vi "子界面-查看某框.vi"(0 "框号":dbl format="%#_13g", 1 "框组":T3(array[cluster]), 2 "临界Z值":i32, 3 "反射图原始路径":path, 4 "临界面积百分比值":dbl, 5 "预先配置的灰度阈值":dbl, 6 "穿透图原始路径":path, 7 "部位信息":string[](array[string])=["", "34.500000", "32.500000", "1121", "34", "54.955926", "分层类", "不合格", ""], 12 "产品规格":cluster{"产品长度（周长）（mm）":dbl, "产品宽度（母线长）（mm）":dbl}) -> (14 "弥散类检测结果":string[][](table), 19 "分层类检测结果":string[][](table))   [LabVIEW 2018]
uses:
  <vilib>/vision/NI_Vision_Development_Module.lvlib
panel:
  in  "格式字符串 3":string="%f"
  in  "分隔符（'\\'代码显示） 2":string="\t"
  out "弥散和分层临界灰度值":i64
  out "弥散缺陷个数":i32
  out "分层缺陷个数":i32
  out "合格？ 弥散类":string="fencengThreshold"
  out "合格？分层类":string="fencengThreshold"
  in  "stop":bool caption="停止"
  out "?":T1(plugin-control)
  out "Threshold Image":T1(plugin-control)
  out "Threshold Image":T1(plugin-control)
  out "Threshold Image":T1(plugin-control)
  in  "Tab Control":T2
  out "穿透ROI":T1(plugin-control)
  out "Threshold Image":T1(plugin-control)
  out "?":T1(plugin-control)
  out "?":T1(plugin-control)
  out "Threshold Image":T1(plugin-control)
  out "Threshold Image":T1(plugin-control)
  out "弥散测量结果":dbl[][](array[numeric]) format="%.2f"
  out "?":string
  out "面积 (pixels)":i32
  in  "格式字符串 2":string="%f"
  in  "分隔符（'\\'代码显示）":string="\t"
  out "分层测量结果":dbl[][](array[numeric]) format="%.2f"
  out "缺陷初步分类的临界值":sgl format="%#.3f"
  # "所选区域信息"
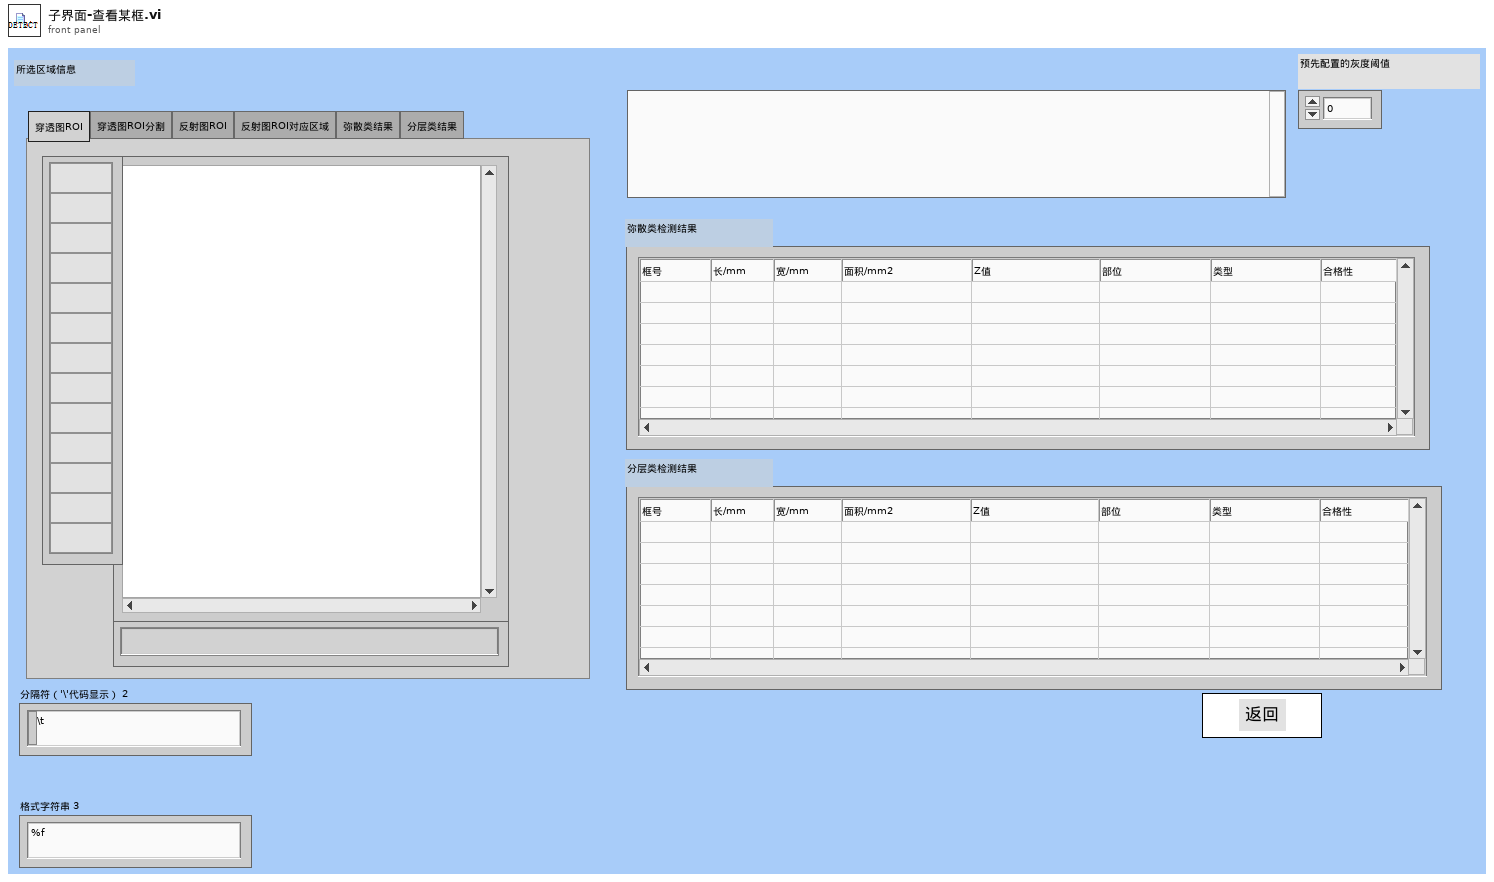
[diagram p1: front panel]
types:
  T1 = typedef "IMAQ Image.ctl" = refnum<image>
  T2 = typedef "控件 1.ctl" = enum32{"穿透图ROI", "穿透图ROI分割", "反射图ROI", "反射图ROI对应区域", "弥散类结果", "分层类结果"}
  T3 = cluster{"Global Rectangle":i32[], "Contours":cluster{"Contour Type":u32, "ROI Type":u32, "Points":i32[]}[]}[]
  T4 = typedef "Image Type" = u32
  T5 = typedef "Particle Parameters" = i32
  T6 = cluster{"Measurement Parameter":T5, "Range Lower Value":dbl, "Range Upper Value":dbl, "Range":bool, "Measurement Type":bool}[]
  T7 = cluster{"Global Rectangle":i32[], "Contours":cluster{"Contour Type":u32, "ROI Type":u32, "Points":i32[]}[]}
  T8 = cluster{"histogram":u32[], "Minimal Value":sgl, "Maximal Value":sgl, "Starting Value":sgl, "Interval Width":sgl, "Mean Value":sgl, "Standard  Variation":sgl, "Area (pixels)":i32}
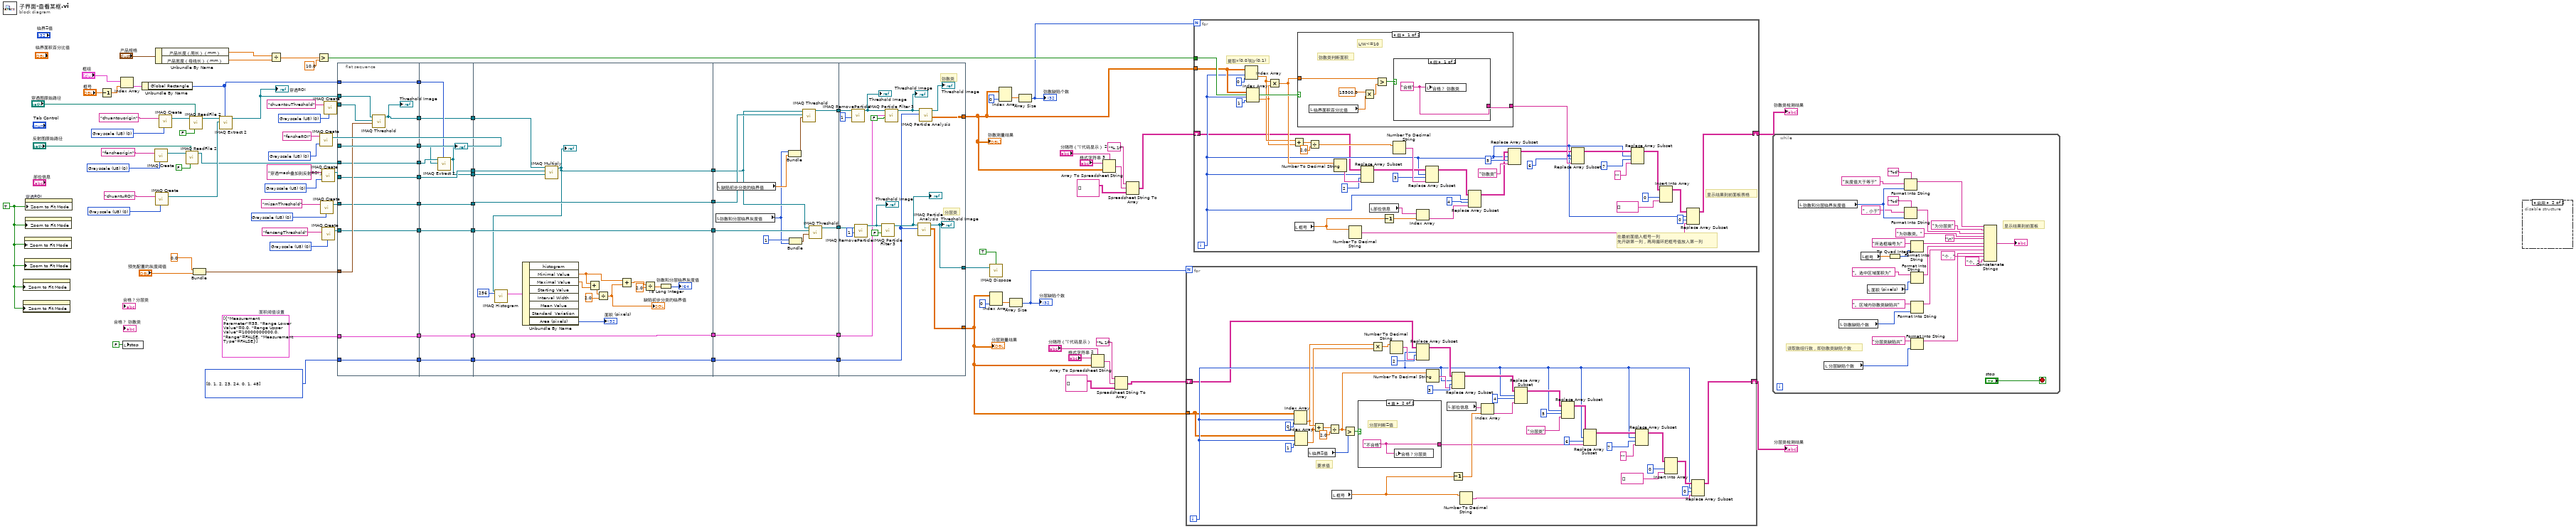
[diagram p0: block diagram]
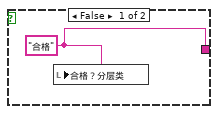
[diagram p2: hidden frame]
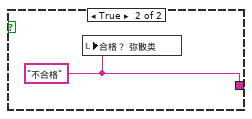
[diagram p3: hidden frame]
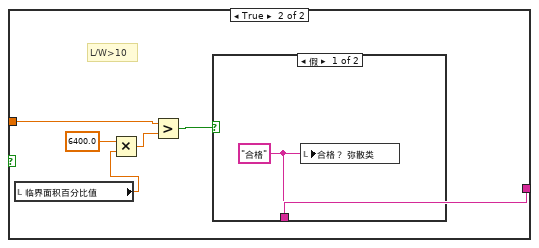
[diagram p4: hidden frame]
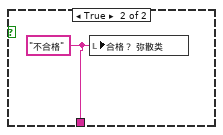
[diagram p5: hidden frame]
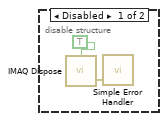
[diagram p6: hidden frame]
diagram:
  w62 = T4 0 items=["Grayscale (U8)", "Grayscale (I16)", "Grayscale (SGL)", "Complex (CSG)", "RGB (U32)", "HSL (U32)", "RGB (U64)", "Grayscale (U16)"] ("Image Type")
  w63 = T4 0 items=["Grayscale (U8)", "Grayscale (I16)", "Grayscale (SGL)", "Complex (CSG)", "RGB (U32)", "HSL (U32)", "RGB (U64)", "Grayscale (U16)"] ("Image Type")
  w64 = T4 0 items=["Grayscale (U8)", "Grayscale (I16)", "Grayscale (SGL)", "Complex (CSG)", "RGB (U32)", "HSL (U32)", "RGB (U64)", "Grayscale (U16)"] ("Image Type")
  w68 = T4 0 items=["Grayscale (U8)", "Grayscale (I16)", "Grayscale (SGL)", "Complex (CSG)", "RGB (U32)", "HSL (U32)", "RGB (U64)", "Grayscale (U16)"] ("Image Type")
  w72 = T4 0 items=["Grayscale (U8)", "Grayscale (I16)", "Grayscale (SGL)", "Complex (CSG)", "RGB (U32)", "HSL (U32)", "RGB (U64)", "Grayscale (U16)"] ("Image Type")
  w22 = i32[] [0, 1, 2, 23, 24, 0, 1, 48] items=["Bounding Rect Width", "Bounding Rect Height", "Area"] ("Pixel Measurements")
  w27 = T6 [{"Measurement Parameter"=35, "Range Lower Value"=0.0, "Range Upper Value"=10000000000.0, "Range"=FALSE, "Measurement Type"=FALSE}]  # 面积阈值设置
  w86 = T4 0 items=["Grayscale (U8)", "Grayscale (I16)", "Grayscale (SGL)", "Complex (CSG)", "RGB (U32)", "HSL (U32)", "RGB (U64)", "Grayscale (U16)"] ("Image Type")
  w55 = T4 0 items=["Grayscale (U8)", "Grayscale (I16)", "Grayscale (SGL)", "Complex (CSG)", "RGB (U32)", "HSL (U32)", "RGB (U64)", "Grayscale (U16)"] ("Image Type")
  w90 = T4 0 items=["Grayscale (U8)", "Grayscale (I16)", "Grayscale (SGL)", "Complex (CSG)", "RGB (U32)", "HSL (U32)", "RGB (U64)", "Grayscale (U16)"] ("Image Type")
  w98 = TRUE ("Zoom to Fit Mode")
  n1 = property class="ImageControl"("Zoom to Fit Mode"=w98) -> ()  [unwired: 2 in, 2 out]
  n2 = property class="ImageControl"("Zoom to Fit Mode"=w98) -> ()  [unwired: 2 in, 2 out]
  n3 = property class="ImageControl"("Zoom to Fit Mode"=w98) -> ()  [unwired: 2 in, 2 out]
  n4 = property class="ImageControl"("Zoom to Fit Mode"=w98) -> ()  [unwired: 2 in, 2 out]
  n5 = property class="ImageControl"("Zoom to Fit Mode"=w98) -> ()  [unwired: 2 in, 2 out]
  n6 = property on="穿透ROI" class="ImageControl"("Zoom to Fit Mode"=w98) -> ()  [unwired: 2 in, 2 out]
  n7 = Decrement(x="框号") -> (x-1=w92:dbl)
  n8 = Index Array(array="框组", index=w92) -> (element=w93:T7)
  n9 = local write "stop"(FALSE ("stop")) -> ()
  n10 = Unbundle By Name(w93) -> ("Global Rectangle"=w54:i32[])
  n11 = call "IMAQ Create"("Image Name"="fansheorigin", "Image Type"=w68) -> ("New Image"=w67:T1)  [unwired: 3 in, 1 out]
  n12 = call "IMAQ Create"("Image Name"="chuantuROI", "Image Type"=w72) -> ("New Image"=w71:T1)  [unwired: 3 in, 1 out]
  n13 = Unbundle By Name("产品规格") -> ("产品长度（周长）（mm）"=w80:dbl, "产品宽度（母线长）（mm）"=w79:dbl)
  n14 = call "IMAQ Create"("Image Name"="chuantouorigin", "Image Type"=w90) -> ("New Image"=w74:T1)  [unwired: 3 in, 1 out]
  n15 = call "IMAQ ReadFile 2"("Use File Path Image Type"=FALSE, "File Path"="反射图原始路径", "Image"=w67) -> ("Image Out"=w50:T1)  [unwired: 4 in, 4 out]
  n16 = call "IMAQ ReadFile 2"("Use File Path Image Type"=FALSE, "File Path"="穿透图原始路径", "Image"=w74) -> ("Image Out"=w75:T1)  [unwired: 4 in, 4 out]
  n17 = Bundle(0.0, "预先配置的灰度阈值"="预先配置的灰度阈值") -> (w17:cluster{dbl, "预先配置的灰度阈值":dbl})  [unwired: 1 in]
  n18 = call "IMAQ Extract 2"("Optional Rectangle"=w54, "Image Dst"=w71, "Image Src"=w75) -> ("Image Dst Out"=w52:T1)  [unwired: 7 in, 1 out]
  "穿透ROI" <- w52
  n19 = Divide(x=w80, y=w79) -> (x/y=w83:dbl)
  n20 = Greater?(x=w83, y=10.0) -> (0:w78:bool)
  n21 = call "IMAQ Create"("Image Name"="fansheROI", "Image Type"=w55) -> ("New Image"=w51:T1)  [unwired: 3 in, 1 out]
  n22 = call "IMAQ Create"("Image Name"="misanThreshold", "Image Type"=w62) -> ("New Image"=w37:T1)  [unwired: 3 in, 1 out]
  n23 = call "IMAQ Create"("Image Name"="穿透mask叠加到反射ROI上", "Image Type"=w86) -> ("New Image"=w45:T1)  [unwired: 3 in, 1 out]
  n24 = call "IMAQ Create"("Image Name"="fencengThreshold", "Image Type"=w63) -> ("New Image"=w35:T1)  [unwired: 3 in, 1 out]
  n25 = call "IMAQ Create"("Image Name"="chuantouThreshold", "Image Type"=w64) -> ("New Image"=w53:T1)  [unwired: 3 in, 1 out]
  n26 = flat-sequence {
    tunnel: w54 -> [w110]
    tunnel: w53 -> [w109]
    tunnel: w52 -> [w108]
    tunnel: w17 -> [w107]
    tunnel: w51 -> [w106]
    tunnel: w50 -> [w105]
    tunnel: [w110] -> w49
    tunnel: [w106] -> w48
    tunnel: [w105] -> w47
    tunnel: [w104] -> w46
    tunnel: w45 -> [w104]
    tunnel: [w103] -> w42
    tunnel: w37 -> [w102]
    tunnel: [w102] -> w39
    tunnel: [w101] -> w36
    tunnel: w35 -> [w101]
    tunnel: [w100] -> w28
    tunnel: w27 -> [w100]
    tunnel: [w99] -> w23
    tunnel: w22 -> [w99]
    tunnel: w49 -> [w120]
    tunnel: w48 -> [w111]
    tunnel: w47 -> [w112]
    tunnel: w46 -> [w119]
    tunnel: [w119] -> w44
    tunnel: [w118] -> w43
    tunnel: w42 -> [w118]
    tunnel: [w117] -> w41
    tunnel: w39 -> [w116]
    tunnel: [w116] -> w38
    tunnel: w36 -> [w115]
    tunnel: [w115] -> w34
    tunnel: w28 -> [w114]
    tunnel: [w114] -> w26
    tunnel: w23 -> [w113]
    tunnel: [w113] -> w21
    tunnel: w44 -> [w140]
    tunnel: w43 -> [w139]
    tunnel: w41 -> [w138]
    tunnel: [w137] -> w40
    tunnel: w38 -> [w137]
    tunnel: w34 -> [w136]
    tunnel: [w136] -> w33
    tunnel: [w131] -> w32
    tunnel: w26 -> [w130]
    tunnel: [w130] -> w25
    tunnel: w21 -> [w129]
    tunnel: [w129] -> w20
    tunnel: w40 -> [w152]
    tunnel: w33 -> [w151]
    tunnel: w32 -> [w150]
    tunnel: [w149] -> w30
    tunnel: [w148] -> w29
    tunnel: w25 -> [w147]
    tunnel: [w147] -> w24
    tunnel: w20 -> [w146]
    tunnel: [w146] -> w19
    tunnel: [w163] -> w3
    tunnel: [w158] -> w11
    tunnel: [w157] -> w31
    tunnel: w30 -> [w156]
    tunnel: w29 -> [w155]
    tunnel: w24 -> [w154]
    tunnel: w19 -> [w153]
    frame #0 {
      n27 = call "IMAQ Threshold"("Range"=w107, "Image Dst"=w109, "Image Src"=w108) -> ("Image Dst Out"=w103:T1)  [unwired: 3 in, 5 out]
      "Threshold Image" <- w103
    }
    frame #1 {
      n28 = call "IMAQ Extract 2"("Optional Rectangle"=w120, "Image Dst"=w111, "Image Src"=w112) -> ("Image Dst Out"=w117:T1)  [unwired: 7 in, 1 out]
      "?" <- w117
    }
    frame #2 {
      n29 = call "IMAQ Multiply"("Image Src A"=w139, "Image Dst"=w140, "Image Src B"=w138) -> ("Image Dst Out"=w131:T1)  [unwired: 4 in, 1 out]
      "?" <- w131
      n30 = call "IMAQ Histogram"("Number of Classes"=256, "Image"=w131) -> ("Histogram Report"=w134:T8)  [unwired: 8 in, 1 out]
      n31 = Unbundle By Name(w134) -> ("Minimal Value"=w123:sgl, "Maximal Value"=w125:sgl, "Area (pixels)"=→"面积 (pixels)":i32)  [unwired: 5 out]
      n32 = Add(x=w123, y=w125) -> (x+y=w124:sgl)
      n33 = Divide(x=w124, y=sgl 2.0) -> (x/y=w122:sgl)
      "缺陷初步分类的临界值" <- w122
      n34 = Add(x=w123, y=w122) -> (x+y=w121:sgl)
      n35 = Divide(x=w121, y=sgl 2.0) -> (x/y=w126:sgl)
      n36 = To Long Integer(number=w126) -> (32bit integer=→"弥散和分层临界灰度值":i32)
    }
    frame #3 {
      n37 = local read "弥散和分层临界灰度值"() -> (w142:i64)
      n38 = local read "缺陷初步分类的临界值"() -> (w144:sgl)
      n39 = Bundle("弥散和分层临界灰度值"=w142, "缺陷初步分类的临界值"=w144) -> (w145:cluster{"弥散和分层临界灰度值":i64, "缺陷初步分类的临界值":sgl})  [unwired: 1 in]
      n40 = Bundle(1, "弥散和分层临界灰度值"=w142) -> (w141:cluster{i32, "弥散和分层临界灰度值":i64})  [unwired: 1 in]
      n41 = call "IMAQ Threshold"("Range"=w145, "Image Dst"=w152, "Image Src"=w150) -> ("Image Dst Out"=w148:T1)  [unwired: 3 in, 5 out]
      n42 = call "IMAQ Threshold"("Range"=w141, "Image Dst"=w151, "Image Src"=w150) -> ("Image Dst Out"=w149:T1)  [unwired: 3 in, 5 out]
    }
    frame #4 {
      # "分层类"
      # "弥散类"
      n43 = call "IMAQ RemoveParticle"("Number of Erosion"=1, "Image Src"=w155) -> ("Image Dst Out"=w166:T1)  [unwired: 8 in, 1 out]
      "Threshold Image" <- w166
      n44 = call "IMAQ RemoveParticle"("Number of Erosion"=1, "Image Src"=w156) -> ("Image Dst Out"=w161:T1)  [unwired: 8 in, 1 out]
      "Threshold Image" <- w161
      n45 = call "IMAQ Particle Filter 3"("Image Src"=w161, "Keep/Remove Particles (F)"=FALSE) -> ("Image Dst Out"=w162:T1)  [unwired: 11 in, 2 out]
      "?" <- w162
      n46 = call "IMAQ Particle Filter 3"("Image Src"=w166, "Selection Values"=w154, "Keep/Remove Particles (F)"=FALSE) -> ("Image Dst Out"=w167:T1)  [unwired: 10 in, 2 out]
      "Threshold Image" <- w167
      n47 = call "IMAQ Particle Analysis"("Pixel Measurements"=w153, "Image"=w162) -> ("Particle Measurements (Pixels)"=w158:dbl[][], "Image Out (duplicate)"=w157:T1)  [unwired: 4 in, 4 out]
      "Threshold Image" <- w157
      n48 = call "IMAQ Particle Analysis"("Pixel Measurements"=w153, "Image"=w167) -> ("Particle Measurements (Real-World)"=w163:dbl[][], "Image Out (duplicate)"=→"Threshold Image":T1)  [unwired: 4 in, 4 out]
    }
  }
  n49 = call "IMAQ Dispose"("All Images? (No)"=TRUE, "Image"=w31) -> ()  [unwired: 4 in, 1 out]
  n50 = Index Array(array=w11, index (col)=0 ("禁用的索引 (列)")) -> (element=w60:dbl[])  [unwired: 1 in]
  n51 = Index Array(array=w3, index (col)=0 ("禁用的索引 (列)")) -> (element=w58:dbl[])  [unwired: 1 in]
  n52 = Array Size(array=w60) -> (size(s)=w18:i32)
  "分层缺陷个数" <- w18
  n53 = Array Size(array=w58) -> (size(s)=w77:i32)
  "弥散缺陷个数" <- w77
  n54 = Array To Spreadsheet String(delimiter (Tab)="分隔符（'\\'代码显示）", array=w11, 3:"格式字符串 2") -> (spreadsheet string=w14:string)
  n55 = Array To Spreadsheet String(delimiter (Tab)="分隔符（'\\'代码显示） 2", array=w3, 3:"格式字符串 3") -> (spreadsheet string=w6:string)
  n56 = Spreadsheet String To Array(format string="%.1f", spreadsheet string=w14, array type (2D Dbl)=string[][] [] ("Array")) -> (array=w10:string[][])  [unwired: 1 in]
  n57 = Spreadsheet String To Array(format string="%.1f", spreadsheet string=w6, array type (2D Dbl)=string[][] [] ("Array")) -> (array=w2:string[][])  [unwired: 1 in]
  n58 = for {
    N: w18 -> [_]
    tunnel: w11 -> [w171]
    shift-right: [w169] -> w9
    shift-left: w10 -> [w170]
    i -> [w174]
    # "要求值"
    n59 = Index Array(array=w171, index (row)=w174, index (col)=0 ("禁用的索引 (列)")) -> (element=w187:dbl)
    n60 = Index Array(array=w171, index (row)=w174, index (col)=1 ("禁用的索引 (列)")) -> (element=w186:dbl)
    n61 = local read "临界Z值"() -> (w205:i32)
    n62 = Add(x=w187, y=w186) -> (x+y=w207:dbl)
    n63 = Divide(x=w207, y=2.0) -> (x/y=w200:dbl)
    n64 = local read "框号"() -> (w172:dbl)
    n65 = Greater?(x=w200, y=w205) -> (0:w208:bool)
    n66 = case shown="真" w208 {
      tunnel: [w209 w210] -> w180
      frame False {
        w209 = "合格" ("合格？")
        n67 = local write "合格？分层类"(w209) -> ()
      }
      frame True {
        w210 = "不合格" ("合格？")
        # "分层判断Z值"
        n68 = local write "合格？分层类"(w210) -> ()
      }
    }
    n69 = Multiply(x=w187, y=w186) -> (x*y=w198:dbl)
    n70 = Number To Decimal String(number=w198) -> (decimal integer string=w185:string)  [unwired: 1 in]
    n71 = Replace Array Subset(array=w170, new element=w185, index (row)=w174, index (col)=2 ("禁用的索引 (列)")) -> (w194:string[][])
    n72 = Number To Decimal String(number=w200) -> (decimal integer string=w184:string)  [unwired: 1 in]
    n73 = local read "部位信息"() -> (w191:string[])
    n74 = Decrement(x=w172) -> (x-1=w190:dbl)
    n75 = Replace Array Subset(array=w194, new element=w184, index (row)=w174, index (col)=3 ("禁用的索引 (列)")) -> (w189:string[][])
    n76 = Number To Decimal String(number=w172) -> (decimal integer string=w173:string)  [unwired: 1 in]
    n77 = Index Array(array=w191, index=w190) -> (element=w183:string)
    n78 = Replace Array Subset(array=w189, new element=w183, index (row)=w174, index (col)=4 ("禁用的索引 (列)")) -> (w188:string[][])
    n79 = Replace Array Subset(array=w188, new element="分层类" ("新元素/子数组"), index (row)=w174, index (col)=5 ("禁用的索引 (列)")) -> (w193:string[][])
    n80 = Replace Array Subset(array=w193, new element=w180, index (row)=w174, index (col)=6 ("禁用的索引 (列)")) -> (w196:string[][])
    n81 = Replace Array Subset(array=w196, new element="" ("新元素/子数组"), index (row)=w174, index (col)=7 ("禁用的索引 (列)")) -> (w175:string[][])
    n82 = Insert Into Array(array=w175, index (col)=0 ("禁用的索引 (列)"), new element=string[] [] ("新元素/子数组")) -> (w177:string[][])  [unwired: 1 in]
    n83 = Replace Array Subset(array=w177, new element=w173, index (row)=w174, index (col)=0 ("禁用的索引 (列)")) -> (w169:string[][])
  }
  "分层类检测结果" <- w9
  n84 = for {
    N: w77 -> [_]
    tunnel: w78 -> [w249]
    tunnel: w3 -> [w248]
    shift-right: [w211] -> w1
    shift-left: w2 -> [w212]
    i -> [w215]
    # "在最前面插入框号一列\n先开辟第一列，再用循环把框号值放入第一列"
    # "提取x(0,0)和y(0,1)"
    # "显示结果到前面板表格"
    n85 = Index Array(array=w248, index (row)=w215, index (col)=0 ("禁用的索引 (列)")) -> (element=w237:dbl)
    n86 = Index Array(array=w248, index (row)=w215, index (col)=1 ("禁用的索引 (列)")) -> (element=w236:dbl)
    n87 = Multiply(x=w237, y=w236) -> (x*y=w240:dbl)
    n88 = Add(x=w237, y=w236) -> (x+y=w239:dbl)
    n89 = local read "框号"() -> (w219:dbl)
    n90 = case shown="假" w249 {
      tunnel: w240 -> [w255 w263]
      tunnel: [w253 w261] -> w247
      frame False {
        # "弥散类判断面积"
        # "L/W<=10"
        n91 = local read "临界面积百分比值"() -> (w251:dbl)
        n92 = Multiply(x=15500.0, y=w251) -> (x*y=w250:dbl)
        n93 = Greater?(x=w255, y=w250) -> (0:w254:bool)
        n94 = case shown="假" w254 {
          tunnel: [w256 w257] -> w253
          frame False {
            w256 = "合格" ("合格？")
            n95 = local write "合格？ 弥散类"(w256) -> ()
          }
          frame True {
            w257 = "不合格" ("合格？")
            n96 = local write "合格？ 弥散类"(w257) -> ()
          }
        }
      }
      frame True {
        # "L/W>10"
        n97 = local read "临界面积百分比值"() -> (w258:dbl)
        n98 = Multiply(x=6400.0, y=w258) -> (x*y=w260:dbl)
        n99 = Greater?(x=w263, y=w260) -> (0:w262:bool)
        n100 = case shown="假" w262 {
          tunnel: [w264 w265] -> w261
          frame False {
            w264 = "合格" ("合格？")
            n101 = local write "合格？ 弥散类"(w264) -> ()
          }
          frame True {
            w265 = "不合格" ("合格？")
            n102 = local write "合格？ 弥散类"(w265) -> ()
          }
        }
      }
    }
    n103 = Divide(x=w239, y=2.0) -> (x/y=w233:dbl)
    n104 = Number To Decimal String(number=w240) -> (decimal integer string=w242:string)  [unwired: 1 in]
    n105 = Number To Decimal String(number=w219) -> (decimal integer string=w213:string)  [unwired: 1 in]
    n106 = Replace Array Subset(array=w212, new element=w242, index (row)=w215, index (col)=2 ("禁用的索引 (列)")) -> (w228:string[][])
    n107 = local read "部位信息"() -> (w224:string[])
    n108 = Decrement(x=w219) -> (x-1=w223:dbl)
    n109 = Number To Decimal String(number=w233) -> (decimal integer string=w235:string)  [unwired: 1 in]
    n110 = Index Array(array=w224, index=w223) -> (element=w222:string)
    n111 = Replace Array Subset(array=w228, new element=w235, index (row)=w215, index (col)=3 ("禁用的索引 (列)")) -> (w221:string[][])
    n112 = Replace Array Subset(array=w221, new element=w222, index (row)=w215, index (col)=4 ("禁用的索引 (列)")) -> (w220:string[][])
    n113 = Replace Array Subset(array=w220, new element="弥散类" ("新元素/子数组"), index (row)=w215, index (col)=5 ("禁用的索引 (列)")) -> (w227:string[][])
    n114 = Replace Array Subset(array=w227, new element=w247, index (row)=w215, index (col)=6 ("禁用的索引 (列)")) -> (w226:string[][])
    n115 = Replace Array Subset(array=w226, new element="" ("新元素/子数组"), index (row)=w215, index (col)=7 ("禁用的索引 (列)")) -> (w218:string[][])
    n116 = Insert Into Array(array=w218, index (col)=0 ("禁用的索引 (列)"), new element=string[] [] ("新元素/子数组")) -> (w216:string[][])  [unwired: 1 in]
    n117 = Replace Array Subset(array=w216, new element=w213, index (row)=w215, index (col)=0 ("禁用的索引 (列)")) -> (w211:string[][])
  }
  "弥散类检测结果" <- w1
  n118 = while {
    stop <- "stop" stop-if-true
    # "显示结果到前面板"
    # "读取数组行数，即弥散类缺陷个数"
    n119 = local read "弥散和分层临界灰度值"() -> (w292:i64)
    n120 = local read "分层缺陷个数"() -> (w267:i32)
    n121 = local read "弥散缺陷个数"() -> (w266:i32)
    n122 = local read "框号"() -> (w283:dbl)
    n123 = local read "面积 (pixels)"() -> (w286:i32)
    n124 = To Quad Integer(1:w283) -> (0:w284:i64)
    n125 = Format Into String(format string="%d" ("格式字符串"), initial string="灰度值大于等于" ("初始字符串"), w292) -> (resulting string=w288:string)  [unwired: 1 in, 1 out]
    n126 = Format Into String(format string="%d" ("格式字符串"), initial string="，小于" ("初始字符串"), w292) -> (resulting string=w287:string)  [unwired: 1 in, 1 out]
    n127 = Format Into String(initial string="所选框编号为" ("初始字符串"), w284) -> (resulting string=w282:string)  [unwired: 2 in, 1 out]
    n128 = Format Into String(initial string="。选中区域面积为" ("字符串"), w286) -> (resulting string=w289:string)  [unwired: 2 in, 1 out]
    n129 = Format Into String(initial string="。区域内弥散类缺陷共" ("初始字符串"), w266) -> (resulting string=w290:string)  [unwired: 2 in, 1 out]
    n130 = Format Into String(initial string="分层类缺陷共" ("初始字符串"), w267) -> (resulting string=w291:string)  [unwired: 2 in, 1 out]
    n131 = Concatenate Strings(w288, "为分层类" ("初始字符串"), w287, "为弥散类。" ("初始字符串"), "\n", w282, w289, w290, "个，" ("字符串"), w291, "个。" ("字符串")) -> (→"?":string)
  }
  n132 = disable-structure shown="启用" {
    frame Disabled {
      n133 = call "IMAQ Dispose"("All Images? (No)"=TRUE) -> ("error out"=w294:errorcluster)  [unwired: 5 in]
      n134 = call <vilib>:"Simple Error Handler.vi"("error in (no error)"=w294) -> ()  [unwired: 4 in, 5 out]
    }
    frame Enabled {
    }
  }
  "分层测量结果" <- w11
  "弥散测量结果" <- w3
